vi "while.vi"() -> ()   [LabVIEW 2020]
panel:
  in  "Numeric 3":dbl
  in  "stop 2":bool
  in  "milliseconds to wait 2":u32
  in  "°F 2":dbl(slide) scale=-50.0..100.0
  out "Numeric 2":i32
  out "Thermometer (°C) 2":dbl(slide) scale=-50.0..100.0
  in  "Boolean":bool
  out "Thermometer (°C)":dbl(slide) scale=-50.0..100.0
  out "Numeric":i32
  in  "°F":dbl(slide) scale=-50.0..100.0
  in  "milliseconds to wait":u32
  in  "stop":bool
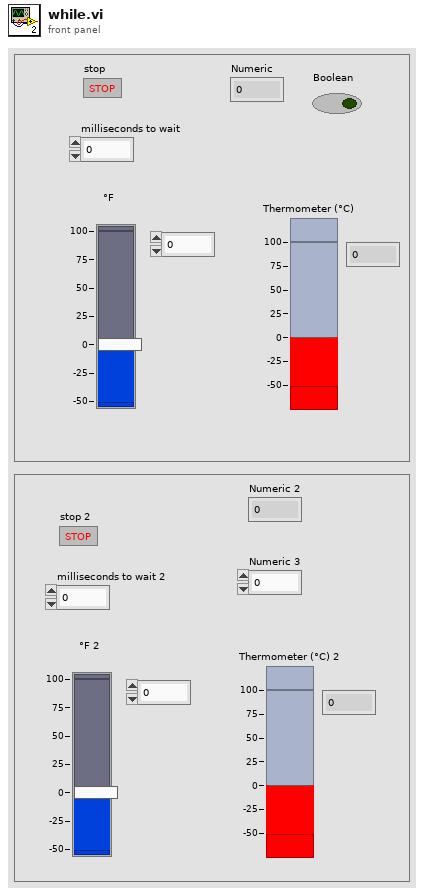
[diagram p1: front panel]
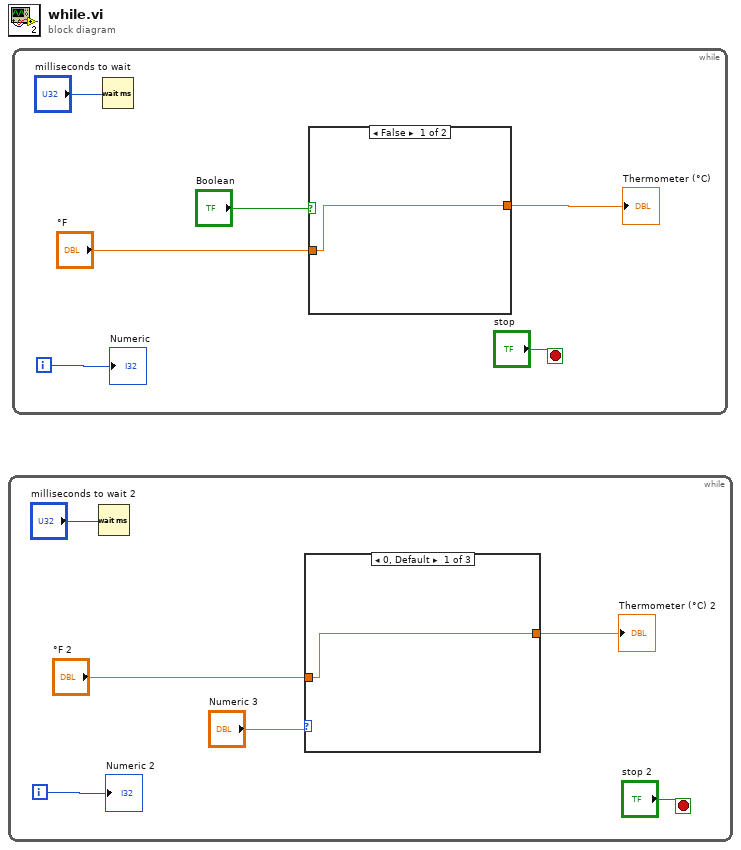
[diagram p0: block diagram]
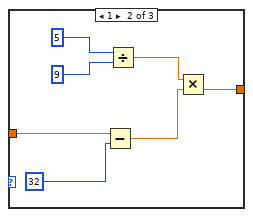
[diagram p2: hidden frame]
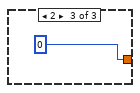
[diagram p3: hidden frame]
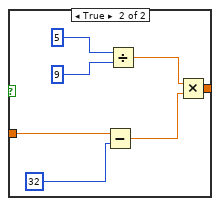
[diagram p4: hidden frame]
diagram:
  n1 = while {
    i -> [w3]
    stop <- "stop 2" stop-if-true
    n2 = Wait (ms)(milliseconds to wait="milliseconds to wait 2") -> ()  [unwired: 1 out]
    n3 = case shown="0, Default" "Numeric 3" {
      tunnel: "°F 2" -> [w7 w12 _]
      tunnel: [w7 w8 0] -> w2
      frame 0, Default {
      }
      frame 1 {
        n4 = Subtract(x=w12, y=32) -> (x-y=w10:dbl)
        n5 = Divide(x=5, y=9) -> (x/y=w9:dbl)
        n6 = Multiply(x=w9, y=w10) -> (x*y=w8:dbl)
      }
      frame 2 {
      }
    }
    "Thermometer (°C) 2" <- w2
    "Numeric 2" <- w3
  }
  n7 = while {
    i -> [w18]
    stop <- "stop" stop-if-true
    n8 = Wait (ms)(milliseconds to wait="milliseconds to wait") -> ()  [unwired: 1 out]
    n9 = case shown="False" "Boolean" {
      tunnel: "°F" -> [w22 w27]
      tunnel: [w22 w23] -> w17
      frame False {
      }
      frame True {
        n10 = Subtract(x=w27, y=32) -> (x-y=w25:dbl)
        n11 = Divide(x=5, y=9) -> (x/y=w24:dbl)
        n12 = Multiply(x=w24, y=w25) -> (x*y=w23:dbl)
      }
    }
    "Thermometer (°C)" <- w17
    "Numeric" <- w18
  }
